vi "Hitronics Dialog - Scan.vi"(5 "error in (no error)":errorcluster) -> (14 "Serial Number":string, 16 "Part Number":string, 17 "Full Scan":string, 18 "Continue Exec?":bool, 19 "error out":errorcluster)   [LabVIEW 2020]
panel:
  out "PN Index":i32
  in  "STOP":bool
  in  "Raw Scan":string
  # "Scan the Hitronics Laser QR Label, then hit the <ENTER> key"
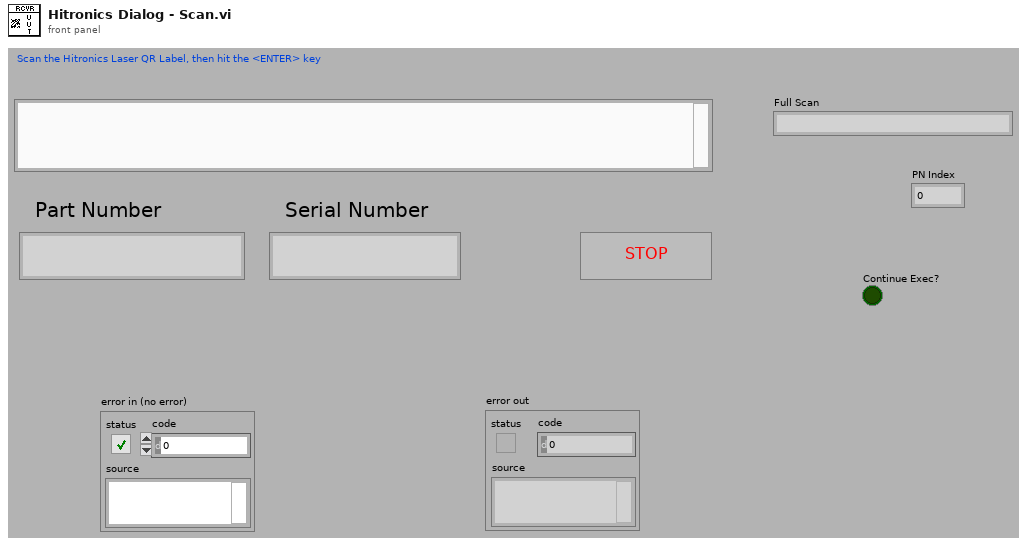
[diagram p1: front panel]
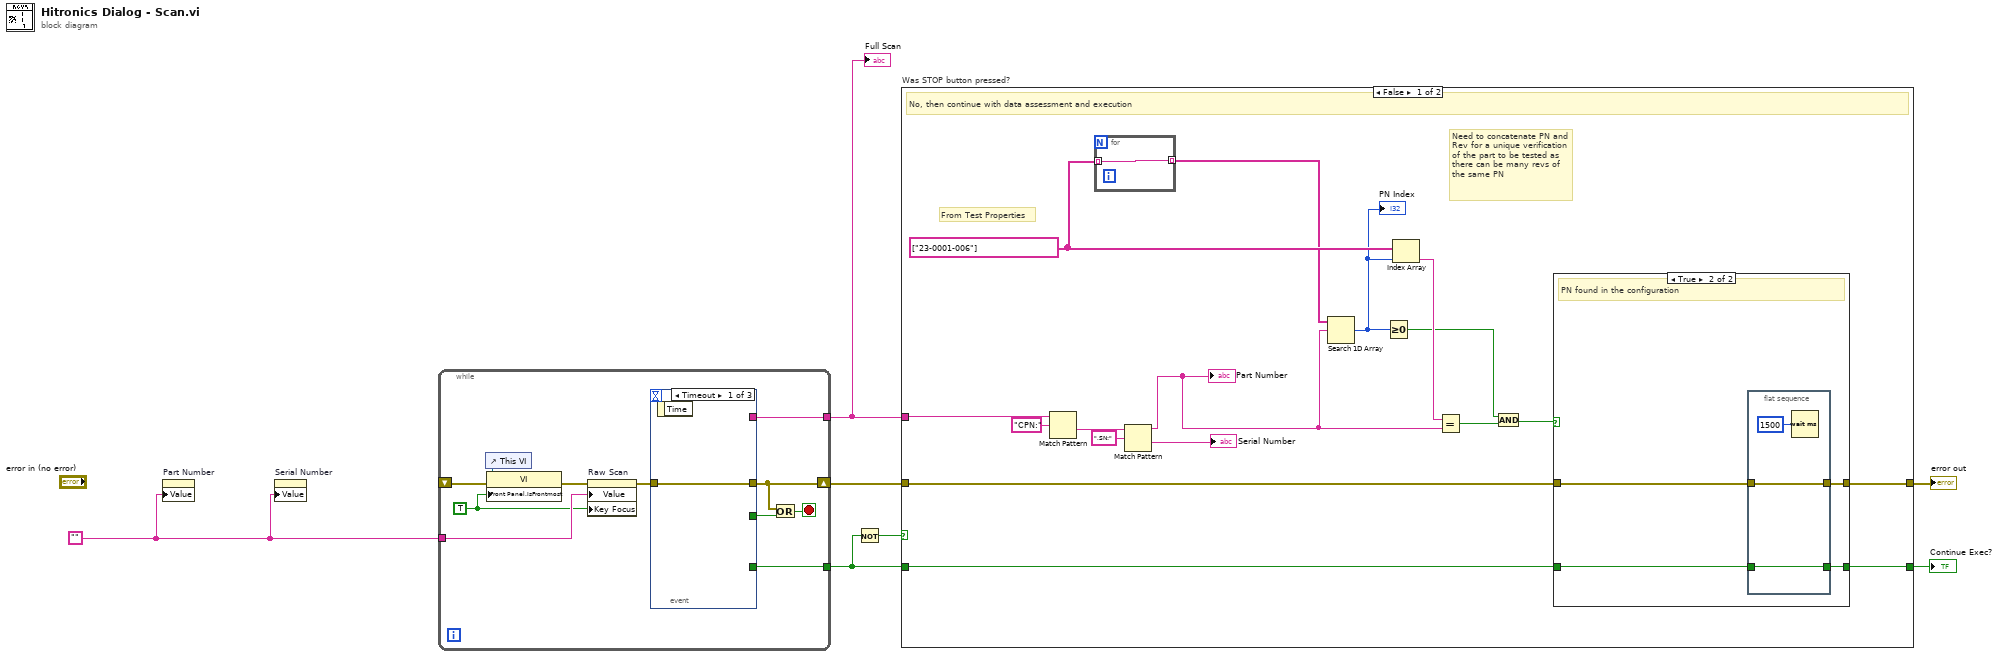
[diagram p0: block diagram]
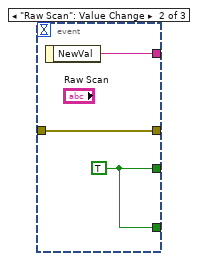
[diagram p2: hidden frame]
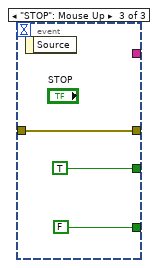
[diagram p3: hidden frame]
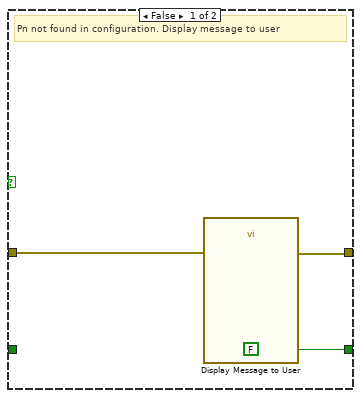
[diagram p4: hidden frame]
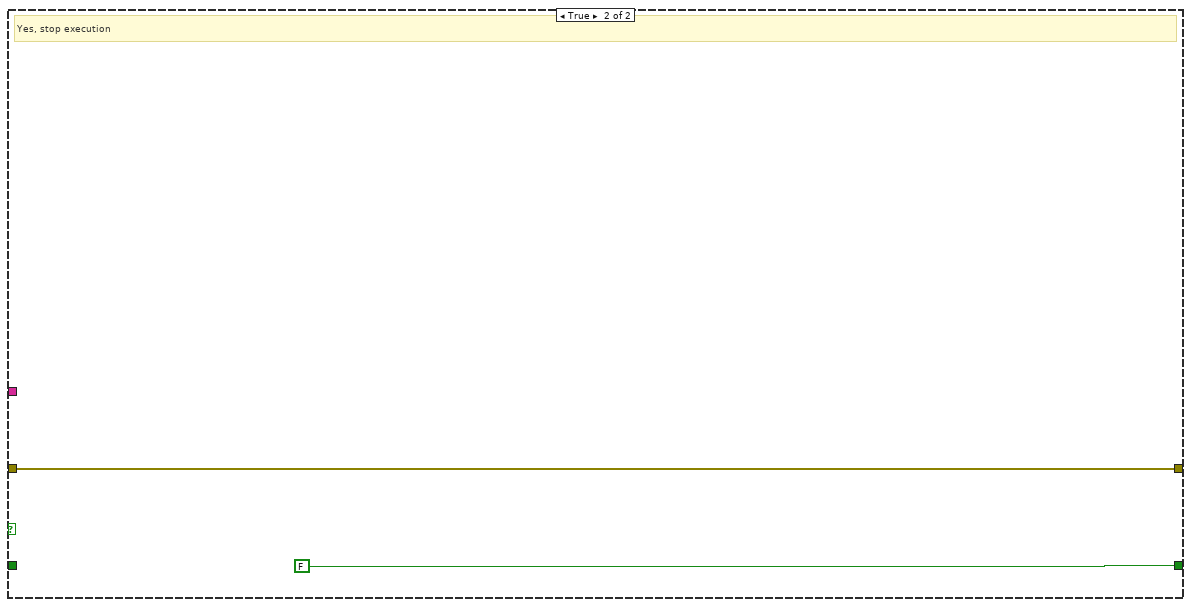
[diagram p5: hidden frame]
diagram:
  w1 = ""
  n1 = property on="Part Number" class="Str"("Value"=w1) -> ()  [unwired: 2 in, 2 out]
  n2 = property on="Serial Number" class="Str"("Value"=w1) -> ()  [unwired: 2 in, 2 out]
  n3 = while {
    shift-right: [w18] -> w7
    shift-left: _ -> [w10]
    tunnel: [w15] -> w2
    tunnel: [w14] -> w4
    tunnel: w1 -> [w12]
    stop <- w16 stop-if-true
    w8 = TRUE
    n4 = control-ref of="This VI"() -> (w11:refnum<vi>)
    n5 = property class="VI"(reference=w11, error in=w10, "Front Panel.IsFrontmost"=w8) -> (error out=w9:errorcluster)  [unwired: 1 out]
    n6 = property on="Raw Scan" class="Str"(error in=w9, "Value"=w12, "Key Focus"=w8) -> (error out=w13:errorcluster)  [unwired: 1 in, 1 out]
    n7 = event shown="[0] Timeout" {
      selector: _ -> [_ _ _]
      dyn-events: _ -> [_ _ _]
      timeout: _ -> [_ _ _]
      tunnel: w13 -> [w19 w22 w25]
      tunnel: [w19 w22 w25] -> w18
      tunnel: [_ w21 TRUE] -> w17
      tunnel: [_ w21 FALSE] -> w14
      tunnel: [_ w20 _] -> w15
      event Timeout {
        n8 = event-data() -> ()  [unwired: 1 in, 1 out]
      }
      event "Raw Scan": Value Change {
        w21 = TRUE
        n9 = event-data() -> ("NewVal"=w20:string)  [unwired: 1 in]
      }
      event "STOP": Mouse Up {
        n10 = event-data() -> ()  [unwired: 1 in, 1 out]
      }
    }
    n11 = Or(x=w18, y=w17) -> (x .or. y?=w16:bool)
  }
  "Full Scan" <- w2
  n12 = Not(x=w4) -> (.not. x?=w5:bool)
  n13 = case "Was STOP button pressed?" shown="False" w5 {
    tunnel: w2 -> [w35 _]
    tunnel: [w42 w54] -> w3
    tunnel: w7 -> [w36 w54]
    tunnel: [w41 FALSE] -> w6
    tunnel: w4 -> [w40 _]
    frame False {
      w39 = string[] ["23-0001-006"] ("Configured PNs")
      # "Need to concatenate PN and Rev for a unique verification of the part to be tested as there can be many revs of the same PN"
      # "From Test Properties"
      # "No, then continue with data assessment and execution"
      n14 = Match Pattern(string=w35, regular expression="CPN:") -> (after substring=w33:string)  [unwired: 1 in, 3 out]
      n15 = for {
        tunnel: w39 -> [w53] mode=indexing
        tunnel: [w53] -> w38 mode=indexing
      }
      n16 = Match Pattern(string=w33, regular expression=",SN:") -> (before substring=w31:string, after substring=→"Serial Number":string)  [unwired: 1 in, 2 out]
      "Part Number" <- w31
      n17 = Search 1D Array(1D array=w38, element=w31) -> (index of element=w29:i32)  [unwired: 1 in]
      "PN Index" <- w29
      n18 = Greater Or Equal To 0?(x=w29) -> (x >= 0?=w28:bool)
      n19 = Index Array(array=w39, index=w29) -> (element=w37:string)
      n20 = Equal?(x=w37, y=w31) -> (x = y?=w27:bool)
      n21 = And(x=w28, y=w27) -> (x .and. y?=w26:bool)
      n22 = case shown="True" w26 {
        tunnel: [w43 w49] -> w42
        tunnel: w36 -> [w44 w48]
        tunnel: [FALSE w47] -> w41
        tunnel: w40 -> [_ w46]
        frame False {
          # "Pn not found in configuration. Display message to user"
          n23 = call "Display Message to User"("error in (no error)"=w44) -> ("error out"=w43:errorcluster)  [unwired: 9 in, 1 out]
        }
        frame True {
          # "PN found in the configuration"
          n24 = flat-sequence {
            tunnel: [w51] -> w49
            tunnel: w48 -> [w51]
            tunnel: [w50] -> w47
            tunnel: w46 -> [w50]
            frame #0 {
              n25 = Wait (ms)(milliseconds to wait=u32 1500) -> ()  [unwired: 1 out]
            }
          }
        }
      }
    }
    frame True {
      # "Yes, stop execution"
    }
  }
  "error out" <- w3
  "Continue Exec?" <- w6
